vi "_Definition.vi"() -> (2 "Definition":T1)   [LabVIEW 2020, in "Conditum-Example.lvlib" / "User.lvclass"]
uses:
  User.lvclass
  Conditum/Columns/String/Definition.ctl
  Conditum/Columns/String/String.lvclass
  Conditum/Attributes.ctl
  Conditum/Conditum.lvlib
  Conditum/Columns/Type/Definition.ctl
  Conditum/Columns/Type/Type.lvclass
  Conditum/Columns/String/String Definition.ctl
  Conditum/Columns/Integer/Definition.ctl
  Conditum/Columns/Integer/Integer.lvclass
  Conditum/Columns/Integer/Integer Definition.ctl
  Conditum/Columns/Timestamp/Timestamp.lvclass
  Conditum/Columns/Timestamp/Definition.ctl
  Conditum/Columns/Timestamp/DateTime Definition.ctl
  Conditum/Columns/Boolean/Boolean.lvclass
  Conditum/Columns/Boolean/Definition.ctl
  Conditum/Columns/Boolean/Boolean Definition.ctl
  Game/Game.lvclass
  Conditum/Relation Mapping.ctl
  Conditum/Columns/Relation/Relation Info.ctl
  Conditum/Columns/Entity Collection/Entity Collection.lvclass
  Conditum/Columns/Entity Collection/Collection Definition.ctl
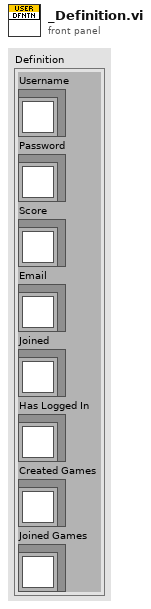
[diagram p1: front panel]
types:
  T1 = cluster{"Username":refnum<class "String.lvclass">, "Password":refnum<class "String.lvclass">, "Score":refnum<class "Integer.lvclass">, "Email":refnum<class "String.lvclass">, "Joined":refnum<class "Timestamp.lvclass">, "Has Logged In":refnum<class "Boolean.lvclass">, "Created Games":refnum<class "Entity Collection.lvclass">, "Joined Games":refnum<class "Entity Collection.lvclass">}
  T2 = typedef "Conditum.lvlib/Columns.lvlib/Entity Collection.lvclass/Collection Definition.ctl" = cluster{"Table Name":string, "Relation":T3}
  T3 = typedef "Conditum.lvlib/Relation Info.ctl" = cluster{"Mapping":T4, "Related To":string, "Reversed By":string}
  T4 = typedef "Conditum.lvlib/Relation Mapping.ctl" = enum16{"OneToMany", "ManyToOne", "ManyToMany", "OneToOne"}
  T5 = typedef "Conditum.lvlib/Columns.lvlib/Boolean.lvclass/Boolean Definition.ctl" = cluster{"Type":T6, "Attributes":T7, "Boolean":T8}
  T6 = typedef "Conditum.lvlib/Columns.lvlib/Type.lvclass/Definition.ctl" = cluster{"Name":string, "Nullable":bool, "Default NULL":bool}
  T7 = typedef "Conditum.lvlib/Attributes.ctl" = cluster{"Primary Key":bool, "Unique":bool, "Foreign Key":bool, "Auto Increment":bool}
  T8 = typedef "Conditum.lvlib/Columns.lvlib/Boolean.lvclass/Definition.ctl" = cluster{"Default":bool}
  T9 = typedef "Conditum.lvlib/Columns.lvlib/Timestamp.lvclass/DateTime Definition.ctl" = cluster{"Type":T6, "Attributes":T7, "DateTime":T10}
  T10 = typedef "Conditum.lvlib/Columns.lvlib/Timestamp.lvclass/Definition.ctl" = cluster{"Default":timestamp}
  T11 = typedef "Conditum.lvlib/Columns.lvlib/String.lvclass/String Definition.ctl" = cluster{"Type":T6, "Attributes":T7, "String":T12}
  T12 = typedef "Conditum.lvlib/Columns.lvlib/String.lvclass/Definition.ctl" = cluster{"Default":string, "Length":i32}
  T13 = typedef "Conditum.lvlib/Columns.lvlib/Integer.lvclass/Integer Definition.ctl" = cluster{"Type":T6, "Attributes":T7, "Integer":T14}
  T14 = typedef "Conditum.lvlib/Columns.lvlib/Integer.lvclass/Definition.ctl" = cluster{"Default":i64}
  T15 = cluster{"String out":refnum<class "String.lvclass">, "String out":refnum<class "String.lvclass">, "Integer out":refnum<class "Integer.lvclass">, "String out":refnum<class "String.lvclass">, "DateTime out":refnum<class "Timestamp.lvclass">, "Boolean out":refnum<class "Boolean.lvclass">, "Entity Collection out":refnum<class "Entity Collection.lvclass">, "Entity Collection out":refnum<class "Entity Collection.lvclass">}
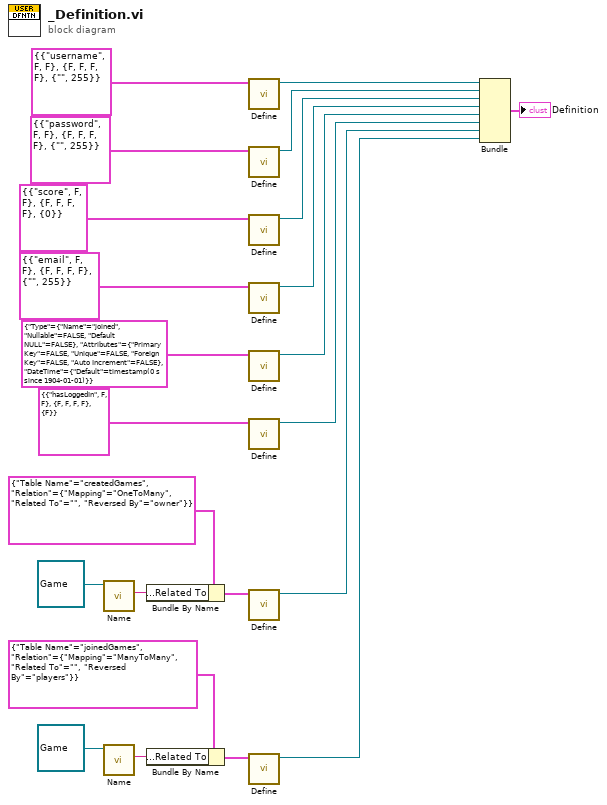
[diagram p0: block diagram]
diagram:
  n1 = call-dynamic "Name.vi"("Entity in"=refnum<class "Game.lvclass"> refnum ("Conditum-Example.lvlib:Game.lvclass")) -> ("Name"=w2:string)  [unwired: 10 in]
  n2 = call-dynamic "Name.vi"("Entity in"=refnum<class "Game.lvclass"> refnum ("Conditum-Example.lvlib:Game.lvclass")) -> ("Name"=w1:string)  [unwired: 10 in]
  n3 = Bundle By Name(cluster=T2 {"Table Name"="createdGames", "Relation"={"Mapping"=enum."OneToMany", "Related To"="", "Reversed By"="owner"}} ("Collection Definition"), "Relation.Related To"=w2) -> (w13:T2)
  n4 = Bundle By Name(cluster=T2 {"Table Name"="joinedGames", "Relation"={"Mapping"=enum."ManyToMany", "Related To"="", "Reversed By"="players"}} ("Collection Definition"), "Relation.Related To"=w1) -> (w5:T2)
  n5 = call "Define.vi"("Definition"=T11 {"Type"={"Name"="username", "Nullable"=FALSE, "Default NULL"=FALSE}, "Attributes"={"Primary Key"=FALSE, "Unique"=FALSE, "Foreign Key"=FALSE, "Auto Increment"=FALSE}, "String"={"Default"="", "Length"=255}}) -> ("String out"=w12:refnum<class "String.lvclass">)  [unwired: 10 in]
  n6 = call "Define.vi"("Definition"=T11 {"Type"={"Name"="password", "Nullable"=FALSE, "Default NULL"=FALSE}, "Attributes"={"Primary Key"=FALSE, "Unique"=FALSE, "Foreign Key"=FALSE, "Auto Increment"=FALSE}, "String"={"Default"="", "Length"=255}}) -> ("String out"=w11:refnum<class "String.lvclass">)  [unwired: 10 in]
  n7 = call "Define.vi"("Integer Definition"=T13 {"Type"={"Name"="score", "Nullable"=FALSE, "Default NULL"=FALSE}, "Attributes"={"Primary Key"=FALSE, "Unique"=FALSE, "Foreign Key"=FALSE, "Auto Increment"=FALSE}, "Integer"={"Default"=0}}) -> ("Integer out"=w10:refnum<class "Integer.lvclass">)  [unwired: 10 in]
  n8 = call "Define.vi"("Definition"=T11 {"Type"={"Name"="email", "Nullable"=FALSE, "Default NULL"=FALSE}, "Attributes"={"Primary Key"=FALSE, "Unique"=FALSE, "Foreign Key"=FALSE, "Auto Increment"=FALSE}, "String"={"Default"="", "Length"=255}}) -> ("String out"=w9:refnum<class "String.lvclass">)  [unwired: 10 in]
  n9 = call "Define.vi"("Definition"=T9 {"Type"={"Name"="joined", "Nullable"=FALSE, "Default NULL"=FALSE}, "Attributes"={"Primary Key"=FALSE, "Unique"=FALSE, "Foreign Key"=FALSE, "Auto Increment"=FALSE}, "DateTime"={"Default"=timestamp(0 s since 1904-01-01)}}) -> ("DateTime out"=w8:refnum<class "Timestamp.lvclass">)  [unwired: 10 in]
  n10 = call "Define.vi"("Init Data"=T5 {"Type"={"Name"="hasLoggedIn", "Nullable"=FALSE, "Default NULL"=FALSE}, "Attributes"={"Primary Key"=FALSE, "Unique"=FALSE, "Foreign Key"=FALSE, "Auto Increment"=FALSE}, "Boolean"={"Default"=FALSE}}) -> ("Boolean out"=w7:refnum<class "Boolean.lvclass">)  [unwired: 10 in]
  n11 = call "Define.vi"("Collection Definition"=w13) -> ("Entity Collection out"=w6:refnum<class "Entity Collection.lvclass">)  [unwired: 10 in]
  n12 = call "Define.vi"("Collection Definition"=w5) -> ("Entity Collection out"=w4:refnum<class "Entity Collection.lvclass">)  [unwired: 10 in]
  n13 = Bundle("String out"=w12, "String out"=w11, "Integer out"=w10, "String out"=w9, "DateTime out"=w8, "Boolean out"=w7, "Entity Collection out"=w6, "Entity Collection out"=w4) -> (→"Definition":T15)  [unwired: 1 in]
